vi "calc_s11.vi"(10 "complex value":dbl[](array[numeric]), 11 "frequency":dbl) -> (3 "s11_data":T1)   [LabVIEW 2025]
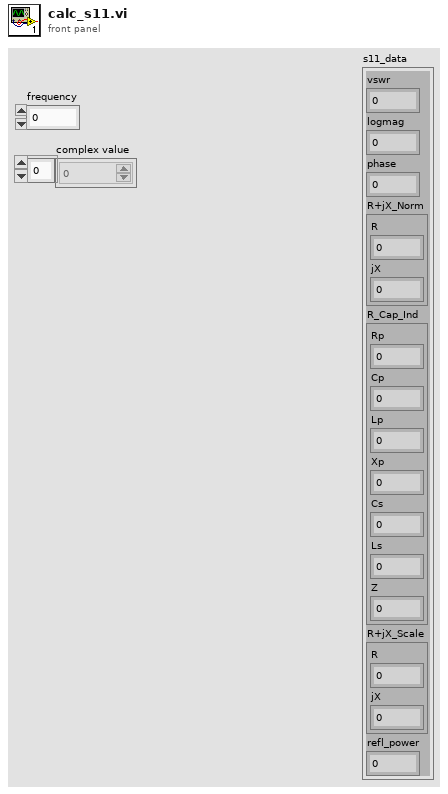
[diagram p1: front panel]
types:
  T1 = cluster{"vswr":dbl, "logmag":dbl, "phase":dbl, "R+jX_Norm":cluster{"R":dbl, "jX":dbl}, "R_Cap_Ind":cluster{"Rp":dbl, "Cp":dbl, "Lp":dbl, "Xp":dbl, "Cs":dbl, "Ls":dbl, "Z":dbl}, "R+jX_Scale":cluster{"R":dbl, "jX":dbl}, "refl_power":dbl}
  T2 = cluster{"Rp":dbl, "Cp":dbl, "Lp":dbl, "Xp":dbl, "Cs":dbl, "Ls":dbl, "Z":dbl}
  T3 = cluster{"vswr":dbl, "logmag":dbl, "phase":dbl, "R+jX_Norm":cluster{"R":dbl, "jX":dbl}, "R_Cap_Ind":cluster{"Rp":dbl, "Cp":dbl, "Lp":dbl, "Xp":dbl, "Cs":dbl, "Ls":dbl, "Z":dbl}, "R+jX_Scale":cluster{"R":dbl, "jX":dbl}, "power":dbl}
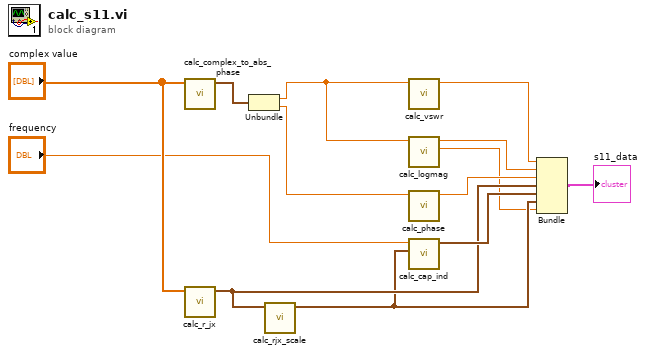
[diagram p0: block diagram]
diagram:
  n1 = call "calc_complex_to_abs_phase.vi"("complex value"="complex value") -> ("output"=w12:cluster{"abs":dbl, "phase":dbl})  [unwired: 10 in]
  n2 = call "calc_r_jx.vi"("complex value"="complex value") -> ("R+jX_Norm"=w4:cluster{"R":dbl, "jX":dbl})  [unwired: 10 in]
  n3 = Unbundle(w12) -> ("abs"=w11:dbl, "phase"=w6:dbl)
  n4 = call "calc_rjx_scale.vi"("R+jX_Norm"=w4) -> ("R+jX_Scale"=w3:cluster{"R":dbl, "jX":dbl})  [unwired: 10 in]
  n5 = call "calc_vswr.vi"("abs"=w11) -> ("vswr"=w9:dbl)  [unwired: 10 in]
  n6 = call "calc_logmag.vi"("abs"=w11) -> ("power"=w2:dbl, "logmag"=w8:dbl)  [unwired: 9 in]
  n7 = call "calc_phase.vi"("phase [rad]"=w6) -> ("phase"=w5:dbl)  [unwired: 10 in]
  n8 = call "calc_cap_ind.vi"("R+jX"=w3, "freq"="frequency") -> ("R_Cap_Ind"=w7:T2)  [unwired: 9 in]
  n9 = Bundle("vswr"=w9, "logmag"=w8, "phase"=w5, "R+jX_Norm"=w4, "R_Cap_Ind"=w7, "R+jX_Scale"=w3, "power"=w2) -> (→"s11_data":T3)  [unwired: 1 in]
